vi "PLC_OP10_Write.vi"(8 "error in (no error)":errorcluster, 11 "S7 Connection in":T1) -> (0 "error out":errorcluster, 3 "S7 Connection out":T1)   [LabVIEW 2017]
uses:
  <vilib>/DATA AHEAD/SP7/typedefs/S7 Connection.ctl
  <vilib>/DATA AHEAD/SP7/typedefs/PLC Type.ctl
  Global/DATA LOG.vi
  <vilib>/DATA AHEAD/SP7/functions/write/write Dint array.vi
  Global/Global 1.vi
  <vilib>/DATA AHEAD/SP7/functions/write/writeString.vi
  <vilib>/DATA AHEAD/SP7/SP7.lvlib
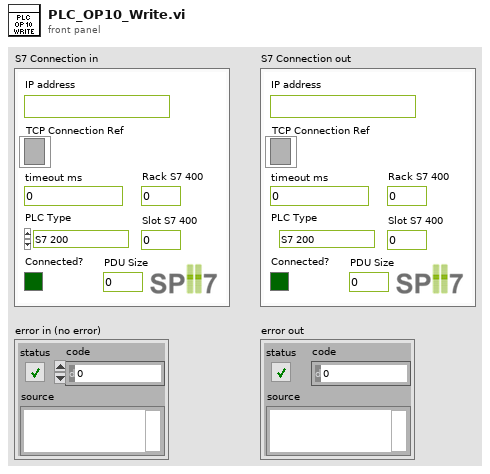
[diagram p1: front panel]
types:
  T1 = typedef "SP7.lvlib/S7 Connection.ctl" = cluster{"TCP Connection Ref":refnum<k5>, "IP address":string, "timeout ms":i32, "Connected?":bool, "PLC Type":T2, "Rack S7 400":u8, "Slot S7 400":u8, "PDU Size":u16, "connection semaphore":T3}
  T2 = typedef "SP7.lvlib/PLC Type.ctl" = enum16{"S7 200", "S7 300/400", "S7 1200", "S7 1500", "LOGO!8"}
  T3 = typedef "Semaphore RefNum" = refnum<k1>
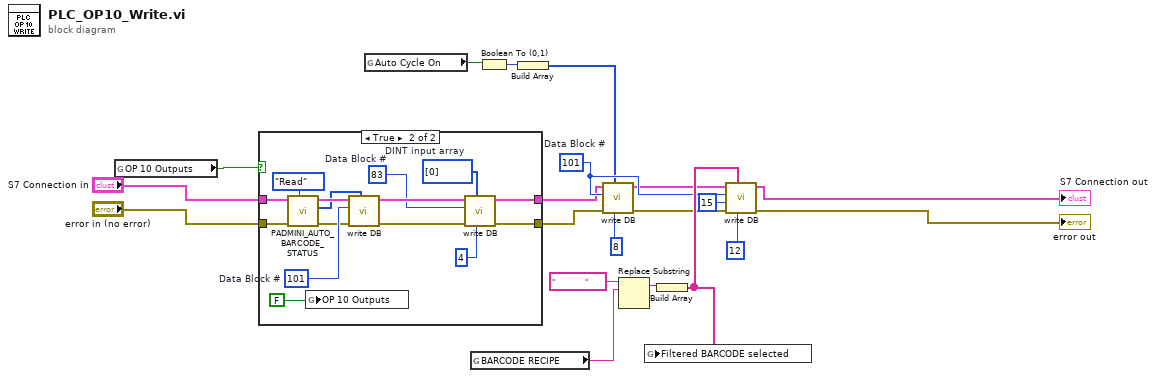
[diagram p0: block diagram]
diagram:
  w14 = u16 101  # Data Block #
  n1 = global read "DATA LOG.vi" "OP 10 Outputs"() -> (w6:bool)
  n2 = case shown="True" w6 {
    tunnel: "S7 Connection in" -> [w21 w35]
    tunnel: [w22 w28] -> w9
    tunnel: [w21 w26] -> w7
    tunnel: "error in (no error)" -> [w22 w32]
    frame False {
    }
    frame True {
      w23 = i32[] [0]  # DINT input array
      w25 = u16 83  # Data Block #
      w36 = u16 101  # Data Block #
      n3 = call "PADMINI_AUTO_BARCODE_STATUS.vi"("Enum"=enum16{"Read", "Write"}."Read", "error in (no error)"=w32) -> ("error out"=w31:errorcluster, "O/P"=w33:i32[])  [unwired: 8 in]
      n4 = global write "DATA LOG.vi" "OP 10 Outputs"(FALSE) -> ()
      n5 = call-poly <vilib>:"write DB.vi"("DINT input array"=w33, "error in (no error)"=w31, "Data Block #"=w36, "S7 Connection in"=w35) -> ("error out"=w29:errorcluster, "S7 Connection out"=w27:T1)  [unwired: 4 in, 2 out]
      n6 = call-poly <vilib>:"write DB.vi"("Item offset [byte]"=u32 4, "DINT input array"=w23, "error in (no error)"=w29, "Data Block #"=w25, "S7 Connection in"=w27) -> ("error out"=w28:errorcluster, "S7 Connection out"=w26:T1)  [unwired: 3 in, 2 out]
    }
  }
  n7 = global read "DATA LOG.vi" "Auto Cycle On"() -> (w3:bool)
  n8 = global read "Global 1.vi" "BARCODE RECIPE"() -> (w17:string)
  n9 = Boolean To (0,1)(Boolean=w3) -> (0, 1=w2:i16)
  n10 = Build Array(w2) -> (w1:i16[])
  n11 = call-poly <vilib>:"write DB.vi"("Item offset [byte]"=u32 8, "DINT input array"=w1, "error in (no error)"=w9, "Data Block #"=w14, "S7 Connection in"=w7) -> ("error out"=w13:errorcluster, "S7 Connection out"=w8:T1)  [unwired: 3 in, 2 out]
  n12 = Replace Substring(4:w17, 5:"               ") -> (1:w18:string)  [unwired: 2 in, 1 out]
  n13 = Build Array(w18) -> (w20:string[])
  n14 = global write "Global 1.vi" "Filtered BARCODE selected"(w20) -> ()
  n15 = call-poly <vilib>:"write DB.vi"("Item offset [byte]"=u32 12, "Input STRINGS"=w20, "error in (no error)"=w13, "String length reserved in DB (default=254)"=u16 15, "Data Block #"=w14, "S7 Connection in"=w8) -> ("error out"=→"error out":errorcluster, "S7 Connection out"=→"S7 Connection out":T1)  [unwired: 2 in, 2 out]
